vi "terminate.vi"(8 "error in (no error)":errorcluster, 11 "StimulatorDL090727DAQmx in":refnum<class "StimulatorDL090727Writer.lvclass">) -> (0 "error out":errorcluster, 3 "StimulatorDL090727DAQmx out":refnum<class "StimulatorDL090727Writer.lvclass">)   [LabVIEW 2010, in "StimulatorDL090727Writer.lvclass"]
uses:
  StimulatorDL090727Writer.lvclass
  StimulatorDL090727Writer.lvclass/StimulatorDL090727Writer.ctl
  SignalWriter/GenericSignalWriter/GenericSignalWriter/GenericSignalWriter.lvclass
  StimulatorDL090724Scaffold/StimulatorDL090724Scaffold/Stimulator090724Scaffold.lvclass
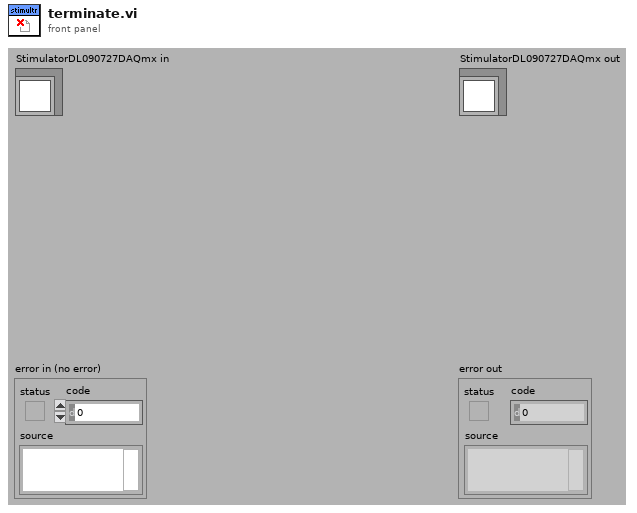
[diagram p1: front panel]
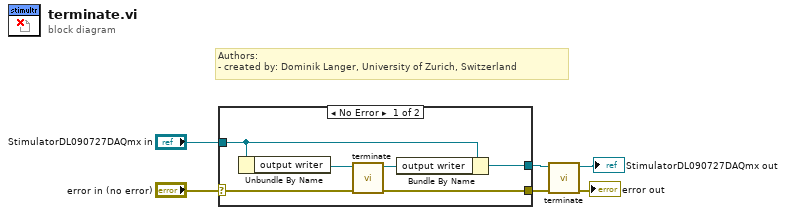
[diagram p0: block diagram]
diagram:
  # "Authors: \n- created by: Dominik Langer, University of Zurich, Switzerland"
  n1 = case shown="No Error" "error in (no error)" {
    selector: "error in (no error)" -> [w8 w14]
    tunnel: [w7 w14] -> w3
    tunnel: [w9 w13] -> w1
    tunnel: "StimulatorDL090727DAQmx in" -> [w10 w13]
    frame No Error {
      n2 = Unbundle By Name(w10) -> ("output writer"=w12:refnum<class "GenericSignalWriter.lvclass">)
      n3 = call-dynamic "terminate.vi"("error in (no error)"=w8, "GenericPlugin in"=w12) -> ("error out"=w7:errorcluster, "GenericPlugin out"=w11:refnum<class "GenericSignalWriter.lvclass">)  [unwired: 8 out]
      n4 = Bundle By Name(cluster=w10, "output writer"=w11) -> (w9:refnum<class "StimulatorDL090727Writer.lvclass">)
    }
    frame Error {
    }
  }
  n5 = call-parent "terminate.vi"("error in (no error)"=w3, "Stimulator090724 in"=w1) -> ("error out"=→"error out":errorcluster, "Stimulator090724 out"=→"StimulatorDL090727DAQmx out":refnum<class "StimulatorDL090727Writer.lvclass">)  [unwired: 8 in]
